vi "ListPara.vi"() -> (3 "Paras":string[](array[string]))   [LabVIEW 2018]
uses:
  <vilib>/Utility/config.llb/NI_LVConfig.lvlib
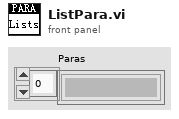
[diagram p1: front panel]
types:
  T1 = typedef "NI_LVConfig.lvlib/Config Data RefNum.ctl" = refnum<k1>
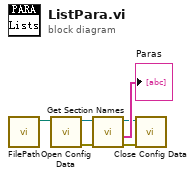
[diagram p0: block diagram]
diagram:
  n1 = call "FilePath.vi"() -> ("添加的路径"=w1:path)  [unwired: 11 in]
  n2 = call <vilib>:"Open Config Data.vi"("configuration file path"=w1) -> ("error out"=w5:errorcluster, "refnum"=w6:T1)  [unwired: 8 in, 1 out]
  n3 = call <vilib>:"Get Section Names.vi"("error in (no error)"=w5, "refnum"=w6) -> ("error out"=w2:errorcluster, "section names"=→"Paras":string[], "refnum out"=w3:T1)  [unwired: 7 in]
  n4 = call <vilib>:"Close Config Data.vi"("error in (no error)"=w2, "refnum"=w3) -> ()  [unwired: 8 in, 2 out]
